vi "Generic command handler.vi"(8 "error in (no error)":errorcluster, 10 "Message in":refnum<class "GenericMessage.lvclass">, 11 "Tomo in":refnum<class "Tomo.lvclass">) -> (0 "error out":errorcluster, 2 "value":string, 3 "Tomo out":refnum<class "Tomo.lvclass">)   [LabVIEW 2012, in "Tomo.lvclass"]
doc: "The generic_command_handler processes the command 'generic'. Commands which are not part of the predefined list of commands fall under the 'generic' command for special activity."
uses:
  Tomo.lvclass
  <vilib>/Distrio/Murmex/GenericMessage/GenericMessage.lvclass
  <vilib>/Distrio/Murmex/Murmex/Murmex.lvclass
  <vilib>/Distrio/Murmex/StartMessage/StartMessage.lvclass
  Current activity.ctl
  file type.ctl
  notice type.ctl
  <vilib>/Distrio/Murmex/StopMessage/StopMessage.lvclass
  <vilib>/Distrio/Murmex/Message/Add or replace parameter.vi
  <vilib>/Distrio/Murmex/Message/Message.lvclass
panel:
  # "This method is called when the GENERIC\ntrigger is sent. \n\nOverride this method when your component needs to\nrespond to this trigger. \n\nCall parent for proper implementation"
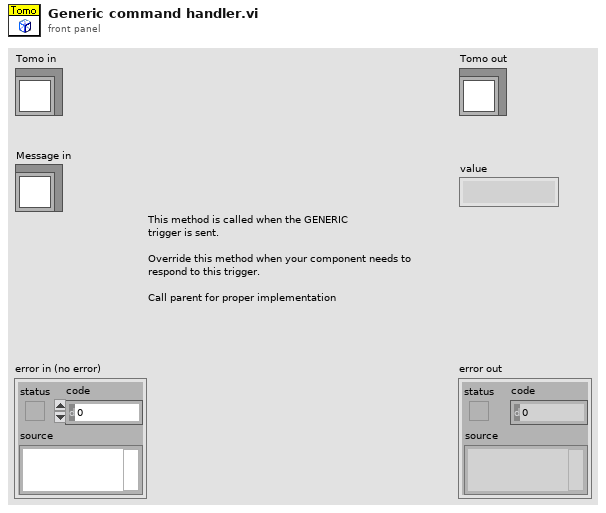
[diagram p1: front panel]
types:
  T1 = typedef "Tomo.lvclass/Current activity.ctl" = enum16{"Idle", "Inter-stack motion", "Autofocus", "Stack acquisition"}
  T2 = typedef "Tomo.lvclass/file type.ctl" = enum16{"Volume map", "Completed stacks"}
  T3 = typedef "Tomo.lvclass/notice type.ctl" = enum16{"Tomography stopped", "Tomography error", "Tomography finished", "Timing issue", "Critical timing issue"}
  T4 = typedef "Tomo.lvclass/volume map.ctl" = enum16{"Cubic volume", "Custom volume", "Self-generate volume"}
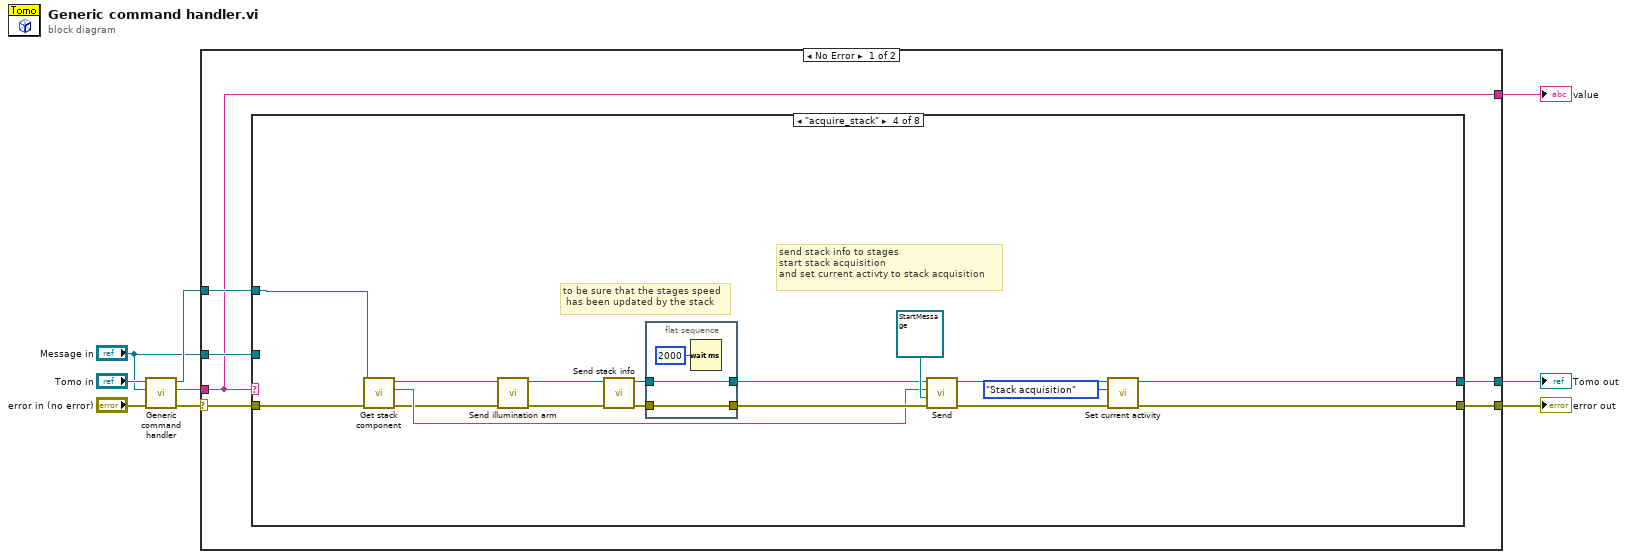
[diagram p0: block diagram]
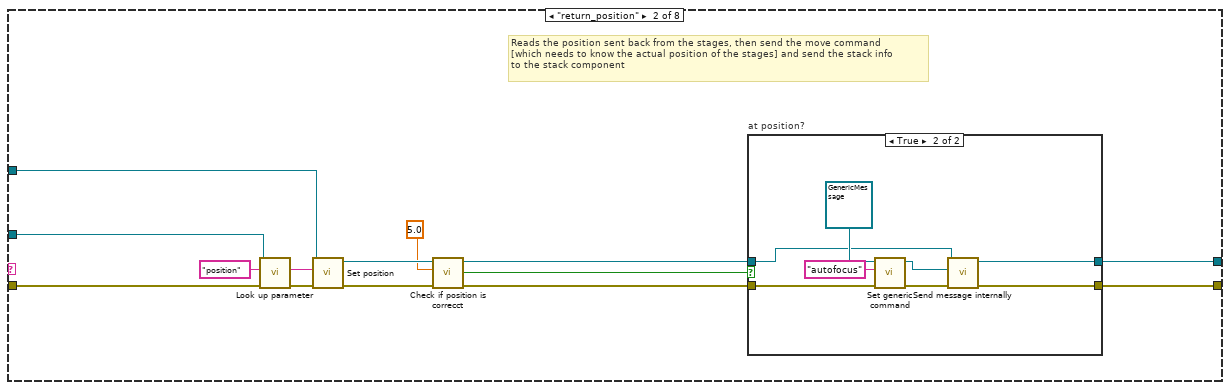
[diagram p3: hidden frame]
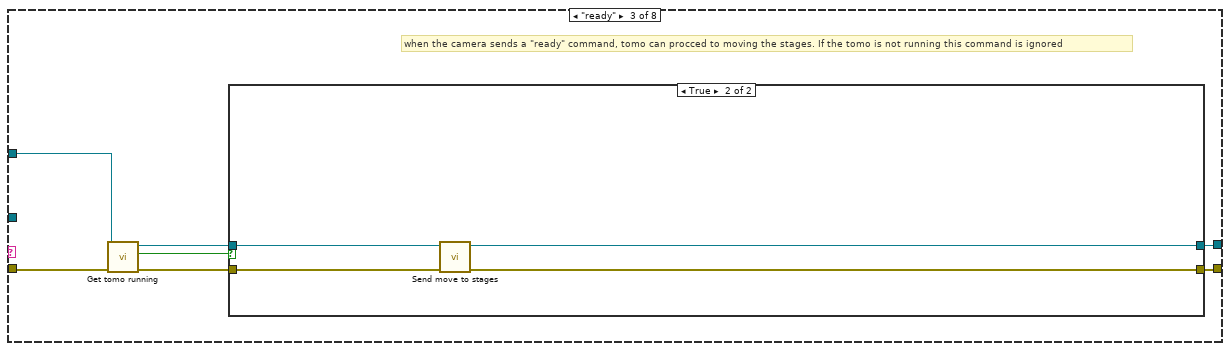
[diagram p5: hidden frame]
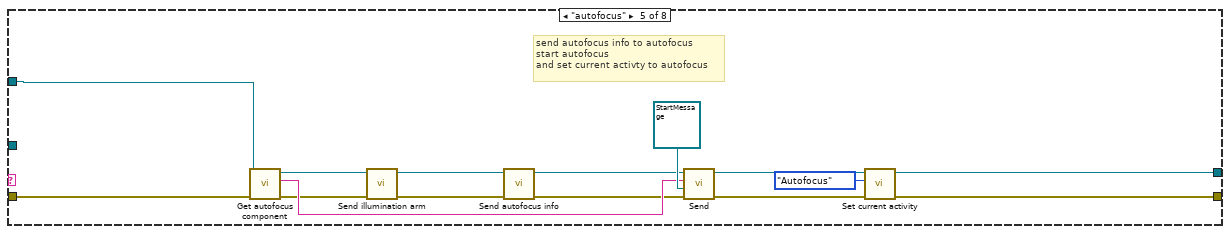
[diagram p7: hidden frame]
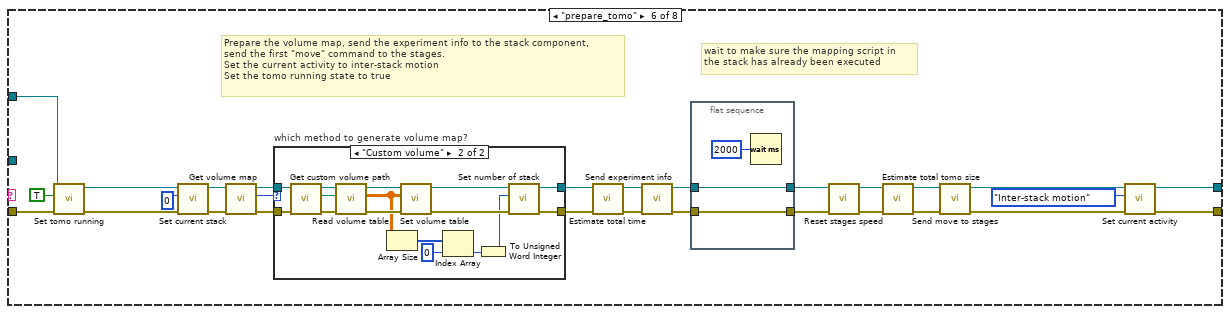
[diagram p8: hidden frame]
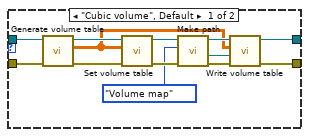
[diagram p9: hidden frame]
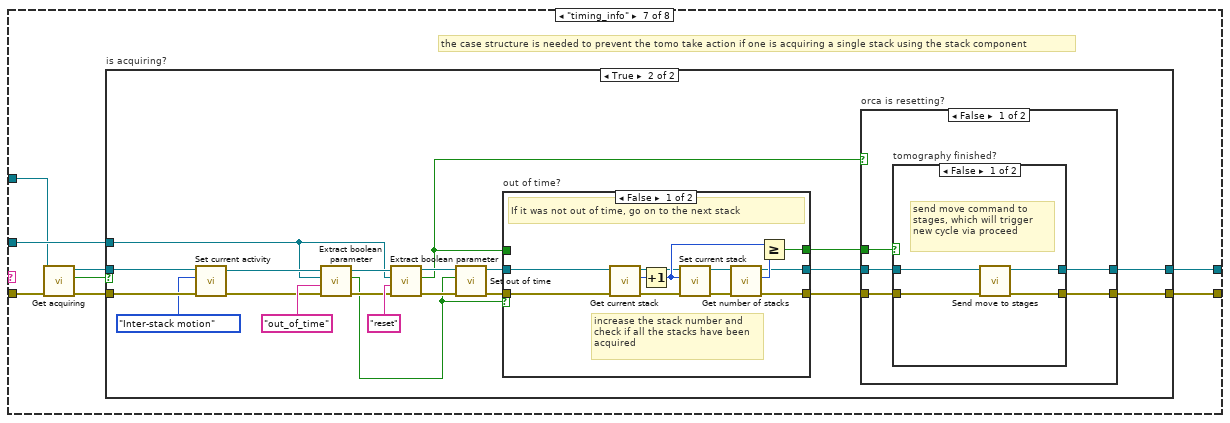
[diagram p10: hidden frame]
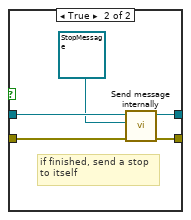
[diagram p12: hidden frame]
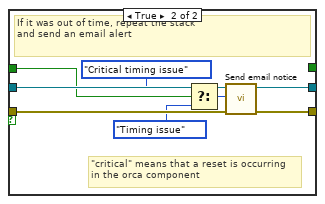
[diagram p14: hidden frame]
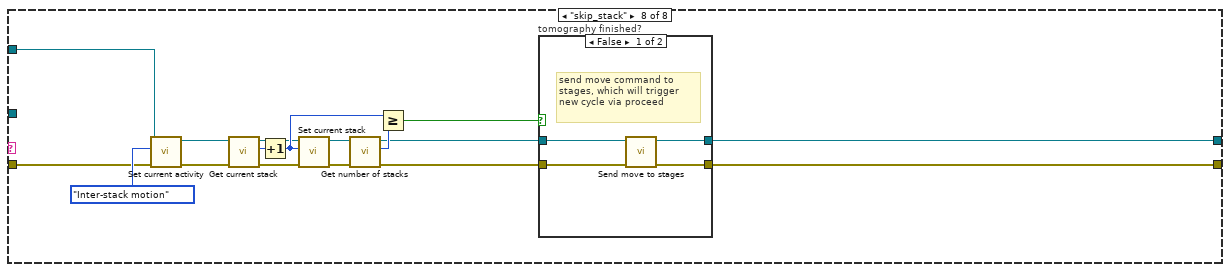
[diagram p15: hidden frame]
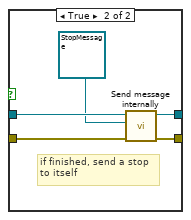
[diagram p16: hidden frame]
diagram:
  n1 = call-parent "Generic command handler.vi"("error in (no error)"="error in (no error)", "Message in"="Message in", "Murmex in"="Tomo in") -> ("error out"=w7:errorcluster, "value"=w6:string, "Murmex out"=w5:refnum<class "Tomo.lvclass">)  [unwired: 6 in]
  n2 = case shown="No Error" w7 {
    selector: w7 -> [w15 w243]
    tunnel: w6 -> [w11 w245]
    tunnel: w5 -> [w14 w244]
    tunnel: "Message in" -> [w13 _]
    tunnel: [w12 w244] -> w3
    tunnel: [w11 w245] -> w2
    tunnel: [w10 w243] -> w1
    frame No Error {
      n3 = case shown="\"acquire_stack\"" w11 {
        tunnel: w15 -> [w17 w31 w48 w66 w82 w94 w154 w232]
        tunnel: w14 -> [w16 w30 w47 w65 w83 w95 w152 w231]
        tunnel: w13 -> [_ w29 _ _ _ _ w157 _]
        tunnel: [w17 w19 w44 w62 w87 w93 w155 w217] -> w10
        tunnel: [w16 w18 w42 w61 w86 w91 w156 w218] -> w12
        frame Default {
        }
        frame "return_position" {
          # "Reads the position sent back from the stages, then send the move command\n[which needs to know the actual position of the stages] and send the stack info\nto the stack component"
          n4 = call <vilib>:"Look up parameter.vi"("error in (no error)"=w31, "name"="position", "Message in"=w29) -> ("error out"=w27:errorcluster, "key"=w26:string)  [unwired: 5 in, 2 out]
          n5 = call-dynamic "Set position.vi"("error in (no error)"=w27, "XML in"=w26, "Tomo in"=w30) -> ("error out"=w25:errorcluster, "Tomo out"=w24:refnum<class "Tomo.lvclass">)  [unwired: 7 in]
          n6 = call-dynamic "Check if position is correcct.vi"("error in (no error)"=w25, "Tolerance (um)"=5.0 ("Tolerance"), "Tomo in"=w24) -> ("error out"=w21:errorcluster, "correct?"=w22:bool, "Tomo out"=w20:refnum<class "Tomo.lvclass">)  [unwired: 6 in]
          n7 = case "at position?" shown="True" w22 {
            tunnel: w21 -> [w33 w40]
            tunnel: w20 -> [w32 w36]
            tunnel: [w33 w35] -> w19
            tunnel: [w32 w34] -> w18
            frame False {
            }
            frame True {
              n8 = call <vilib>:"Set generic command.vi"("error in (no error)"=w40, "generic command"="autofocus", "GenericMessage in"=refnum<class "GenericMessage.lvclass"> refnum ("Distrio Murmex 1.2:GenericMessage")) -> ("error out"=w41:errorcluster, "GenericMessage out"=w37:refnum<class "GenericMessage.lvclass">)  [unwired: 7 in]
              n9 = call <vilib>:"Send message internally.vi"("error in (no error)"=w41, "Message"=w37, "Murmex in"=w36) -> ("error out"=w35:errorcluster, "Murmex out"=w34:refnum<class "Tomo.lvclass">)  [unwired: 7 in]
            }
          }
        }
        frame "ready" {
          # "when the camera sends a \"ready\" command, tomo can procced to moving the stages. If the tomo is not running this command is ignored"
          n10 = call-dynamic "Get tomo running.vi"("error in (no error)"=w48, "Tomo in"=w47) -> ("error out"=w45:errorcluster, "tomo running?"=w46:bool, "Tomo out"=w43:refnum<class "Tomo.lvclass">)  [unwired: 7 in]
          n11 = case shown="True" w46 {
            tunnel: w45 -> [w49 w54]
            tunnel: [w49 w53] -> w44
            tunnel: w43 -> [w50 w52]
            tunnel: [w50 w51] -> w42
            frame False {
            }
            frame True {
              n12 = call-dynamic "Send move to stages.vi"("error in (no error)"=w54, "Tomo in"=w52) -> ("error out"=w53:errorcluster, "Tomo out"=w51:refnum<class "Tomo.lvclass">)  [unwired: 8 in]
            }
          }
        }
        frame "acquire_stack" {
          # "to be sure that the stages speed\n has been updated by the stack"
          # "send stack info to stages\nstart stack acquisition\nand set current activty to stack acquisition"
          n13 = call-dynamic "Get stack component.vi"("error in (no error)"=w66, "Tomo in"=w65) -> ("error out"=w56:errorcluster, "stack component"=w64:string, "Tomo out"=w58:refnum<class "Tomo.lvclass">)  [unwired: 7 in]
          n14 = call-dynamic "Send illumination arm.vi"("error in (no error)"=w56, "Tomo in"=w58) -> ("error out"=w55:errorcluster, "Tomo out"=w57:refnum<class "Tomo.lvclass">)  [unwired: 8 in]
          n15 = call-dynamic "Send stack info.vi"("error in (no error)"=w55, "Tomo in"=w57) -> ("error out"=w67:errorcluster, "Tomo out"=w69:refnum<class "Tomo.lvclass">)  [unwired: 8 in]
          n16 = flat-sequence {
            tunnel: [w74] -> w70
            tunnel: w69 -> [w74]
            tunnel: [w73] -> w68
            tunnel: w67 -> [w73]
            frame #0 {
              n17 = Wait (ms)(milliseconds to wait=u32 2000) -> ()  [unwired: 1 out]
            }
          }
          n18 = call <vilib>:"Send.vi"("error in (no error)"=w68, "Message"=refnum<class "StartMessage.lvclass"> refnum ("Message in"), "recipient"=w64, "Murmex in"=w70) -> ("error out"=w63:errorcluster, "Murmex out"=w60:refnum<class "Tomo.lvclass">)  [unwired: 6 in]
          n19 = call-dynamic "Set current activity.vi"("error in (no error)"=w63, "Current activity"=Current_activity."Stack acquisition", "Tomo in"=w60) -> ("error out"=w62:errorcluster, "Tomo out"=w61:refnum<class "Tomo.lvclass">)  [unwired: 7 in]
        }
        frame "autofocus" {
          # "send autofocus info to autofocus\nstart autofocus\nand set current activty to autofocus"
          n20 = call-dynamic "Get autofocus component.vi"("error in (no error)"=w82, "Tomo in"=w83) -> ("error out"=w76:errorcluster, "autofocus component"=w81:string, "Tomo out"=w78:refnum<class "Tomo.lvclass">)  [unwired: 7 in]
          n21 = call-dynamic "Send illumination arm.vi"("error in (no error)"=w76, "Tomo in"=w78) -> ("error out"=w75:errorcluster, "Tomo out"=w77:refnum<class "Tomo.lvclass">)  [unwired: 8 in]
          n22 = call-dynamic "Send autofocus info.vi"("error in (no error)"=w75, "Tomo in"=w77) -> ("error out"=w79:errorcluster, "Tomo out"=w80:refnum<class "Tomo.lvclass">)  [unwired: 8 in]
          n23 = call <vilib>:"Send.vi"("error in (no error)"=w79, "Message"=refnum<class "StartMessage.lvclass"> refnum ("Message in"), "recipient"=w81, "Murmex in"=w80) -> ("error out"=w88:errorcluster, "Murmex out"=w85:refnum<class "Tomo.lvclass">)  [unwired: 6 in]
          n24 = call-dynamic "Set current activity.vi"("error in (no error)"=w88, "Current activity"=Current_activity."Autofocus", "Tomo in"=w85) -> ("error out"=w87:errorcluster, "Tomo out"=w86:refnum<class "Tomo.lvclass">)  [unwired: 7 in]
        }
        frame "prepare_tomo" {
          # "wait to make sure the mapping script in \nthe stack has already been executed"
          # "Prepare the volume map, send the experiment info to the stack component,\nsend the first \"move\" command to the stages.\nSet the current activity to inter-stack motion\nSet the tomo running state to true"
          n25 = call-dynamic "Set tomo running.vi"("error in (no error)"=w94, "tomo running?"=TRUE, "Tomo in"=w95) -> ("error out"=w100:errorcluster, "Tomo out"=w101:refnum<class "Tomo.lvclass">)  [unwired: 7 in]
          n26 = call-dynamic "Set current stack.vi"("error in (no error)"=w100, "Current stack"=u16 0, "Tomo in"=w101) -> ("error out"=w113:errorcluster, "Tomo out"=w114:refnum<class "Tomo.lvclass">)  [unwired: 7 in]
          n27 = call-dynamic "Get volume map.vi"("error in (no error)"=w113, "Tomo in"=w114) -> ("error out"=w116:errorcluster, "Volume map"=w117:T4, "Tomo out"=w115:refnum<class "Tomo.lvclass">)  [unwired: 7 in]
          n28 = case "which method to generate volume map?" shown="\"Custom volume\"" w117 {
            tunnel: w116 -> [w132 w147]
            tunnel: w115 -> [w133 w145]
            tunnel: [w122 w139] -> w109
            tunnel: [w121 w141] -> w111
            frame "Cubic volume", Default {
              n29 = call-dynamic "Generate volume table.vi"("error in (no error)"=w132, "Tomo in"=w133) -> ("error out"=w130:errorcluster, "Volume table"=w123:dbl[][], "Tomo out"=w131:refnum<class "Tomo.lvclass">)  [unwired: 7 in]
              n30 = call-dynamic "Set volume table.vi"("error in (no error)"=w130, "Volume map in"=w123, "Tomo in"=w131) -> ("error out"=w128:errorcluster, "Tomo out"=w129:refnum<class "Tomo.lvclass">)  [unwired: 7 in]
              n31 = call-dynamic "Make path.vi"("error in (no error)"=w128, "File type"=file_type."Volume map", "Tomo in"=w129) -> ("error out"=w125:errorcluster, "path"=w124:path, "Tomo out"=w126:refnum<class "Tomo.lvclass">)  [unwired: 6 in]
              n32 = call-dynamic "Write volume table.vi"("error in (no error)"=w125, "File name"=w124, "Volume map"=w123, "Tomo in"=w126) -> ("error out"=w121:errorcluster, "Tomo out"=w122:refnum<class "Tomo.lvclass">)  [unwired: 6 in]
            }
            frame "Custom volume" {
              n33 = call-dynamic "Get custom volume path.vi"("error in (no error)"=w147, "Tomo in"=w145) -> ("error out"=w146:errorcluster, "Custom volume path"=w143:path, "Tomo out"=w144:refnum<class "Tomo.lvclass">)  [unwired: 7 in]
              n34 = call "Read volume table.vi"("error in (no error)"=w146, "File path"=w143, "Tomo in"=w144) -> ("error out"=w148:errorcluster, "System Array"=w135:dbl[][], "Tomo out"=w149:refnum<class "Tomo.lvclass">)  [unwired: 6 in]
              n35 = Array Size(array=w135) -> (size(s)=w138:i32[])
              n36 = call-dynamic "Set volume table.vi"("error in (no error)"=w148, "Volume map in"=w135, "Tomo in"=w149) -> ("error out"=w142:errorcluster, "Tomo out"=w140:refnum<class "Tomo.lvclass">)  [unwired: 7 in]
              n37 = Index Array(array=w138, index=0) -> (element=w136:i32)
              n38 = To Unsigned Word Integer(number=w136) -> (unsigned 16bit integer=w134:u16)
              n39 = call-dynamic "Set number of stack.vi"("error in (no error)"=w142, "Number of stacks"=w134, "Tomo in"=w140) -> ("error out"=w141:errorcluster, "Tomo out"=w139:refnum<class "Tomo.lvclass">)  [unwired: 7 in]
            }
          }
          n40 = call-dynamic "Estimate total time.vi"("error in (no error)"=w111, "Tomo in"=w109) -> ("error out"=w110:errorcluster, "Tomo out"=w108:refnum<class "Tomo.lvclass">)  [unwired: 8 in]
          n41 = call-dynamic "Send experiment info.vi"("error in (no error)"=w110, "Tomo in"=w108) -> ("error out"=w96:errorcluster, "Tomo out"=w98:refnum<class "Tomo.lvclass">)  [unwired: 8 in]
          n42 = flat-sequence {
            tunnel: [w120] -> w99
            tunnel: w98 -> [w120]
            tunnel: [w119] -> w97
            tunnel: w96 -> [w119]
            frame #0 {
              n43 = Wait (ms)(milliseconds to wait=u32 2000) -> ()  [unwired: 1 out]
            }
          }
          n44 = call-dynamic "Reset stages speed.vi"("error in (no error)"=w97, "Tomo in"=w99) -> ("error out"=w103:errorcluster, "Tomo out"=w102:refnum<class "Tomo.lvclass">)  [unwired: 8 in]
          n45 = call "Estimate total tomo size.vi"("error in (no error)"=w103, "Tomo in"=w102) -> ("error out"=w106:errorcluster, "Tomo out"=w105:refnum<class "Tomo.lvclass">)  [unwired: 7 in, 1 out]
          n46 = call-dynamic "Send move to stages.vi"("error in (no error)"=w106, "Tomo in"=w105) -> ("error out"=w107:errorcluster, "Tomo out"=w92:refnum<class "Tomo.lvclass">)  [unwired: 8 in]
          n47 = call-dynamic "Set current activity.vi"("error in (no error)"=w107, "Current activity"=Current_activity."Inter-stack motion", "Tomo in"=w92) -> ("error out"=w93:errorcluster, "Tomo out"=w91:refnum<class "Tomo.lvclass">)  [unwired: 7 in]
        }
        frame "timing_info" {
          # "the case structure is needed to prevent the tomo take action if one is acquiring a single stack using the stack component"
          n48 = call-dynamic "Get acquiring.vi"("error in (no error)"=w154, "Tomo in"=w152) -> ("error out"=w153:errorcluster, "is acquiring?"=w150:bool, "Tomo out"=w151:refnum<class "Tomo.lvclass">)  [unwired: 7 in]
          n49 = case "is acquiring?" shown="True" w150 {
            tunnel: w157 -> [_ w162]
            tunnel: [w159 w178] -> w156
            tunnel: [w158 w177] -> w155
            tunnel: w153 -> [w158 w173]
            tunnel: w151 -> [w159 w172]
            frame False {
            }
            frame True {
              n50 = call-dynamic "Set current activity.vi"("error in (no error)"=w173, "Current activity"=Current_activity."Inter-stack motion", "Tomo in"=w172) -> ("error out"=w160:errorcluster, "Tomo out"=w164:refnum<class "Tomo.lvclass">)  [unwired: 7 in]
              n51 = call-dynamic "Extract boolean parameter.vi"("error in (no error)"=w160, "parameter"="out_of_time" ("name"), "Message in"=w162, "Tomo in"=w164) -> ("error out"=w166:errorcluster, "parameter"=w165:bool, "Tomo out"=w163:refnum<class "Tomo.lvclass">)  [unwired: 5 in]
              n52 = call-dynamic "Extract boolean parameter.vi"("error in (no error)"=w166, "parameter"="reset" ("name"), "Message in"=w162, "Tomo in"=w163) -> ("error out"=w170:errorcluster, "parameter"=w168:bool, "Tomo out"=w169:refnum<class "Tomo.lvclass">)  [unwired: 5 in]
              n53 = call-dynamic "Set out of time.vi"("error in (no error)"=w170, "out of time?"=w165, "Tomo in"=w169) -> ("error out"=w175:errorcluster, "Tomo out"=w174:refnum<class "Tomo.lvclass">)  [unwired: 7 in]
              n54 = case "out of time?" shown="False" w165 {
                tunnel: w175 -> [w201 w215]
                tunnel: w174 -> [w200 w216]
                tunnel: [w199 w214] -> w180
                tunnel: [w198 w213] -> w179
                tunnel: [w197 _] -> w176
                tunnel: w168 -> [_ w210]
                frame False {
                  # "increase the stack number and\ncheck if all the stacks have been\nacquired"
                  # "If it was not out of time, go on to the next stack"
                  n55 = call-dynamic "Get current stack.vi"("error in (no error)"=w201, "Tomo in"=w200) -> ("error out"=w203:errorcluster, "Current stack"=w204:u16, "Tomo out"=w202:refnum<class "Tomo.lvclass">)  [unwired: 7 in]
                  n56 = Increment(x=w204) -> (x+1=w208:u16)
                  n57 = call-dynamic "Set current stack.vi"("error in (no error)"=w203, "Current stack"=w208, "Tomo in"=w202) -> ("error out"=w205:errorcluster, "Tomo out"=w206:refnum<class "Tomo.lvclass">)  [unwired: 7 in]
                  n58 = call-dynamic "Get number of stacks.vi"("error in (no error)"=w205, "Tomo in"=w206) -> ("error out"=w199:errorcluster, "Number of stacks"=w207:u16, "Tomo out"=w198:refnum<class "Tomo.lvclass">)  [unwired: 7 in]
                  n59 = Greater Or Equal?(x=w208, y=w207) -> (x >= y?=w197:bool)
                }
                frame True {
                  # "\"critical\" means that a reset is occurring\nin the orca component"
                  # "If it was out of time, repeat the stack\nand send an email alert"
                  n60 = Select(t=notice_type."Critical timing issue" ("Notice type"), s=w210, f=notice_type."Timing issue" ("Notice type")) -> (s? t:f=w209:T3)
                  n61 = call-dynamic "Send email notice.vi"("error in (no error)"=w215, "Notice type"=w209, "Tomo in"=w216) -> ("error out"=w214:errorcluster, "Tomo out"=w213:refnum<class "Tomo.lvclass">)  [unwired: 7 in]
                }
              }
              n62 = case "orca is resetting?" shown="False" w168 {
                tunnel: w180 -> [w185 w196]
                tunnel: w179 -> [w184 w195]
                tunnel: [w183 w195] -> w178
                tunnel: [w182 w196] -> w177
                tunnel: w176 -> [w181 _]
                frame False {
                  n63 = case "tomography finished?" shown="False" w181 {
                    tunnel: w185 -> [w189 w194]
                    tunnel: w184 -> [w188 w191]
                    tunnel: [w187 w192] -> w183
                    tunnel: [w186 w193] -> w182
                    frame False {
                      # "send move command to stages, which will trigger new cycle via proceed"
                      n64 = call-dynamic "Send move to stages.vi"("error in (no error)"=w189, "Tomo in"=w188) -> ("error out"=w186:errorcluster, "Tomo out"=w187:refnum<class "Tomo.lvclass">)  [unwired: 8 in]
                    }
                    frame True {
                      # "if finished, send a stop\nto itself"
                      n65 = call <vilib>:"Send message internally.vi"("error in (no error)"=w194, "Message"=refnum<class "StopMessage.lvclass"> refnum ("Message in"), "Murmex in"=w191) -> ("error out"=w193:errorcluster, "Murmex out"=w192:refnum<class "Tomo.lvclass">)  [unwired: 7 in]
                    }
                  }
                }
                frame True {
                  # "do nothing. Orca will tell\nyou when it's ready"
                }
              }
            }
          }
        }
        frame "skip_stack" {
          n66 = call-dynamic "Set current activity.vi"("error in (no error)"=w232, "Current activity"=Current_activity."Inter-stack motion", "Tomo in"=w231) -> ("error out"=w222:errorcluster, "Tomo out"=w223:refnum<class "Tomo.lvclass">)  [unwired: 7 in]
          n67 = call-dynamic "Get current stack.vi"("error in (no error)"=w222, "Tomo in"=w223) -> ("error out"=w225:errorcluster, "Current stack"=w226:u16, "Tomo out"=w224:refnum<class "Tomo.lvclass">)  [unwired: 7 in]
          n68 = Increment(x=w226) -> (x+1=w230:u16)
          n69 = call-dynamic "Set current stack.vi"("error in (no error)"=w225, "Current stack"=w230, "Tomo in"=w224) -> ("error out"=w227:errorcluster, "Tomo out"=w228:refnum<class "Tomo.lvclass">)  [unwired: 7 in]
          n70 = call-dynamic "Get number of stacks.vi"("error in (no error)"=w227, "Tomo in"=w228) -> ("error out"=w220:errorcluster, "Number of stacks"=w229:u16, "Tomo out"=w219:refnum<class "Tomo.lvclass">)  [unwired: 7 in]
          n71 = Greater Or Equal?(x=w230, y=w229) -> (x >= y?=w221:bool)
          n72 = case "tomography finished?" shown="False" w221 {
            tunnel: w220 -> [w237 w242]
            tunnel: w219 -> [w236 w239]
            tunnel: [w235 w240] -> w218
            tunnel: [w234 w241] -> w217
            frame False {
              # "send move command to stages, which will trigger new cycle via proceed"
              n73 = call-dynamic "Send move to stages.vi"("error in (no error)"=w237, "Tomo in"=w236) -> ("error out"=w234:errorcluster, "Tomo out"=w235:refnum<class "Tomo.lvclass">)  [unwired: 8 in]
            }
            frame True {
              # "if finished, send a stop\nto itself"
              n74 = call <vilib>:"Send message internally.vi"("error in (no error)"=w242, "Message"=refnum<class "StopMessage.lvclass"> refnum ("Message in"), "Murmex in"=w239) -> ("error out"=w241:errorcluster, "Murmex out"=w240:refnum<class "Tomo.lvclass">)  [unwired: 7 in]
            }
          }
        }
      }
    }
    frame Error {
    }
  }
  "error out" <- w1
  "Tomo out" <- w3
  "value" <- w2
